vi "gemm_extended_kalman_filter.vi"(8 "Pin":T1, 9 "Uin":dbl[](array[numeric]), 10 "Xin":dbl[](array[numeric]), 11 "Zin":dbl[](array[numeric])) -> (2 "Pout":T1, 3 "Xout":dbl[](array[numeric]))   [LabVIEW 2013]
uses:
  <vilib>/Analysis/Matrix/Datatypes/RealMatrix.ctl
  <vilib>/Analysis/baseanly.llb/A x Vector.vi
  <vilib>/Analysis/baseanly.llb/Real A x B.vi
  <vilib>/Analysis/_algsub.llb/Real PseudoInverse Matrix.vi
  <vilib>/Analysis/BLAS.llb/dgemm - General Matrix-Matrix Product (DBL).vi
  <vilib>/Analysis/NI_AALPro.lvlib
  <vilib>/Analysis/NI_AALBase.lvlib
  <vilib>/Analysis/Matrix/NI_Matrix.lvlib
  <vilib>/Analysis/NI_AALBLAS.lvlib
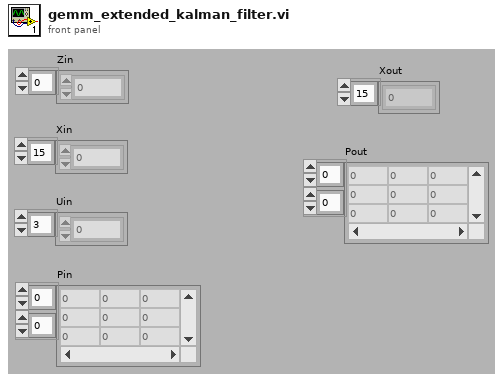
[diagram p1: front panel]
types:
  T1 = typedef "NI_Matrix.lvlib/RealMatrix.ctl" = dbl[][]
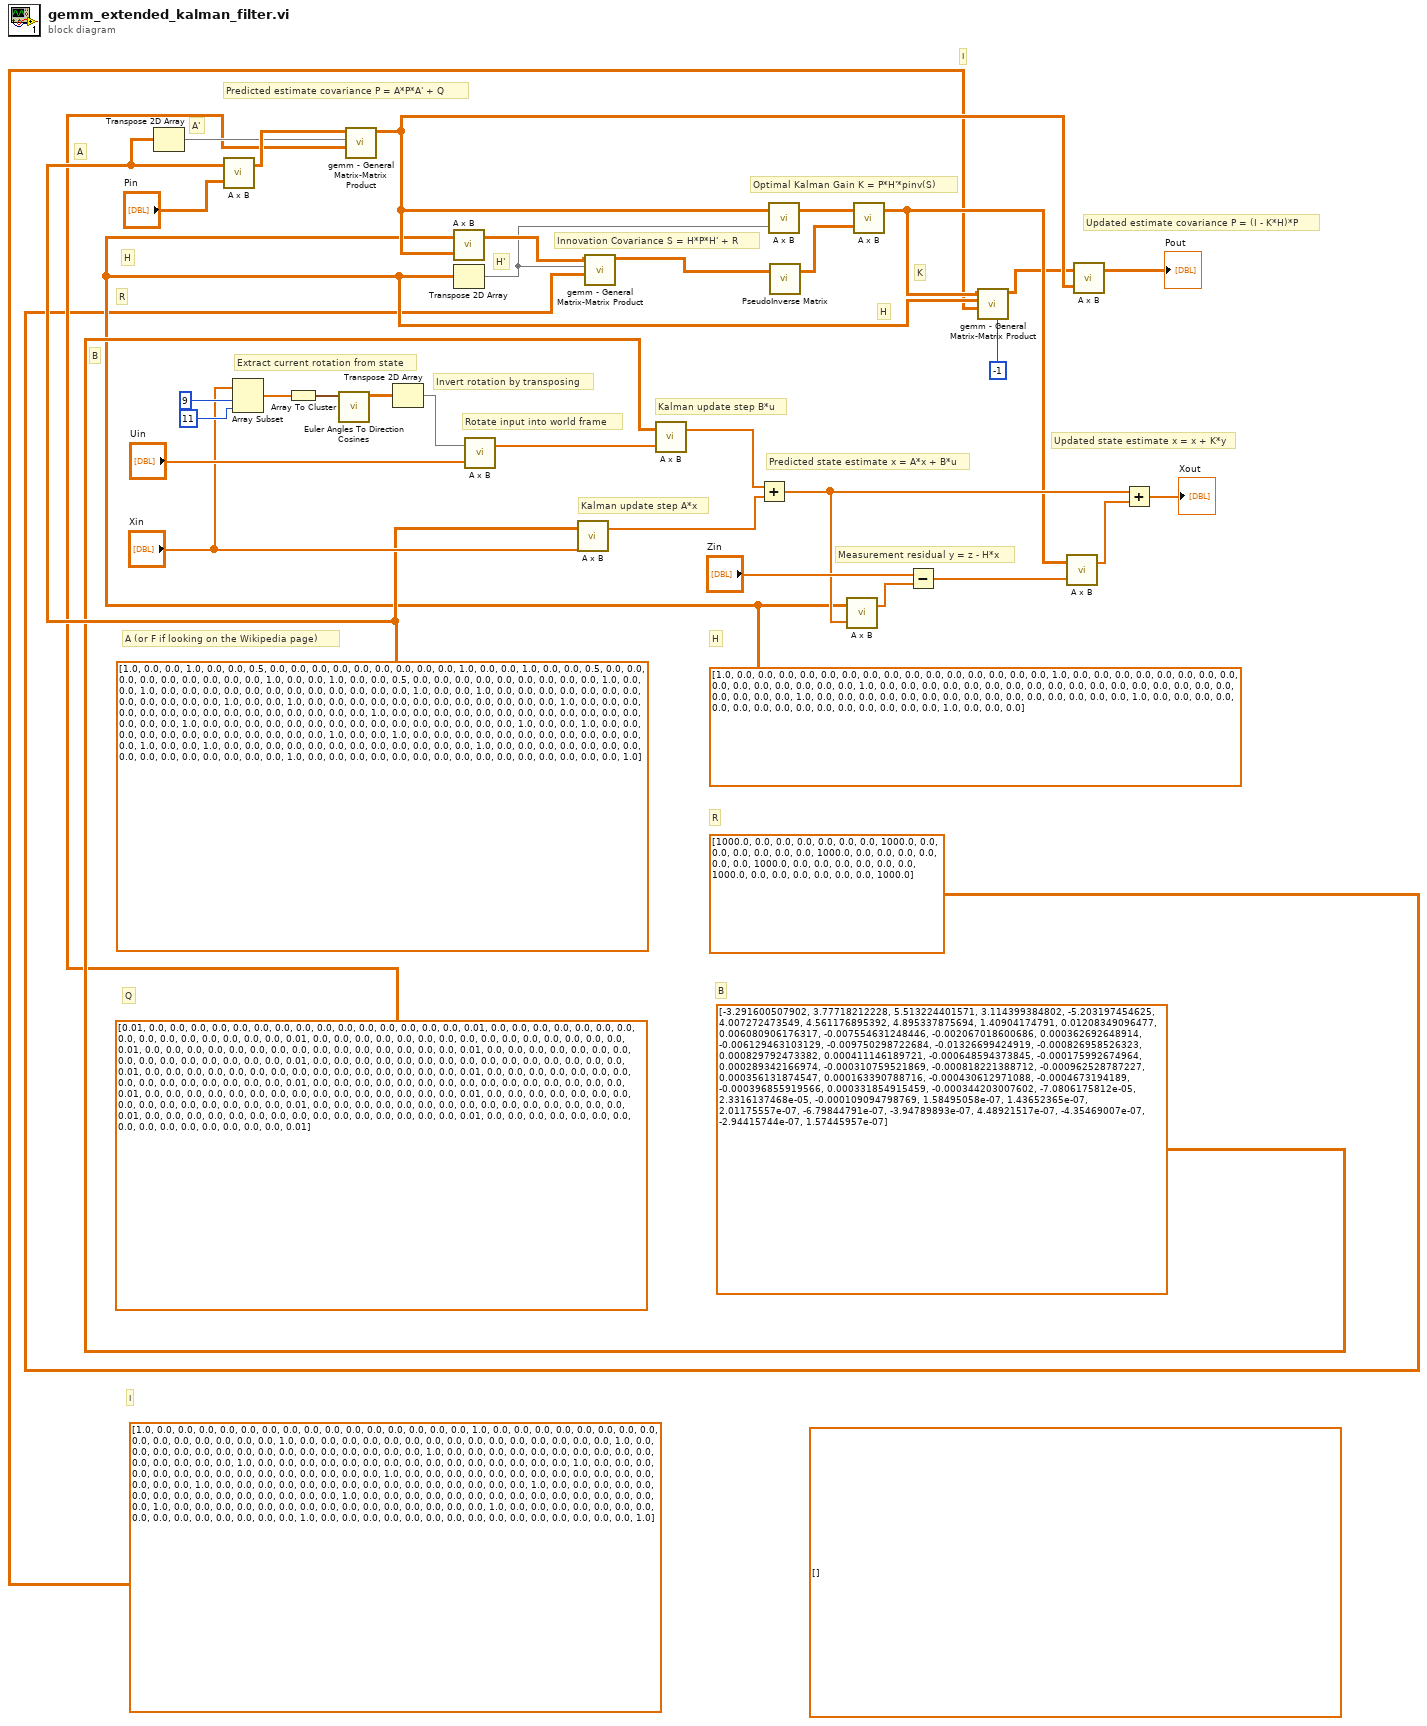
[diagram p0: block diagram]
diagram:
  (unwired) T1 [] ("A + B")
  w8 = T1 [[1.0, 0.0, 0.0, 0.0, 0.0, 0.0, 0.0, 0.0, 0.0, 0.0, 0.0, 0.0, 0.0, 0.0, 0.0], [0.0, 1.0, 0.0, 0.0, 0.0, 0.0, 0.0, 0.0, 0.0, 0.0, 0.0, 0.0, 0.0, 0.0, 0.0], [0.0, 0.0, 1.0, 0.0, 0.0, 0.0, 0.0, 0.0, 0.0, 0.0, 0.0, 0.0, 0.0, 0.0, 0.0], [0.0, 0.0, 0.0, 0.0, 0.0, 0.0, 0.0, 0.0, 0.0, 1.0, 0.0, 0.0, 0.0, 0.0, 0.0], [0.0, 0.0, 0.0, 0.0, 0.0, 0.0, 0.0, 0.0, 0.0, 0.0, 1.0, 0.0, 0.0, 0.0, 0.0], [0.0, 0.0, 0.0, 0.0, 0.0, 0.0, 0.0, 0.0, 0.0, 0.0, 0.0, 1.0, 0.0, 0.0, 0.0]] ("A + B")
  w15 = T1 [[1.0, 0.0, 0.0, 1.0, 0.0, 0.0, 0.5, 0.0, 0.0, 0.0, 0.0, 0.0, 0.0, 0.0, 0.0], [0.0, 1.0, 0.0, 0.0, 1.0, 0.0, 0.0, 0.5, 0.0, 0.0, 0.0, 0.0, 0.0, 0.0, 0.0], [0.0, 0.0, 1.0, 0.0, 0.0, 1.0, 0.0, 0.0, 0.5, 0.0, 0.0, 0.0, 0.0, 0.0, 0.0], [0.0, 0.0, 0.0, 1.0, 0.0, 0.0, 1.0, 0.0, 0.0, 0.0, 0.0, 0.0, 0.0, 0.0, 0.0], [0.0, 0.0, 0.0, 0.0, 1.0, 0.0, 0.0, 1.0, 0.0, 0.0, 0.0, 0.0, 0.0, 0.0, 0.0], [0.0, 0.0, 0.0, 0.0, 0.0, 1.0, 0.0, 0.0, 1.0, 0.0, 0.0, 0.0, 0.0, 0.0, 0.0], [0.0, 0.0, 0.0, 0.0, 0.0, 0.0, 1.0, 0.0, 0.0, 0.0, 0.0, 0.0, 0.0, 0.0, 0.0], [0.0, 0.0, 0.0, 0.0, 0.0, 0.0, 0.0, 1.0, 0.0, 0.0, 0.0, 0.0, 0.0, 0.0, 0.0], [0.0, 0.0, 0.0, 0.0, 0.0, 0.0, 0.0, 0.0, 1.0, 0.0, 0.0, 0.0, 0.0, 0.0, 0.0], [0.0, 0.0, 0.0, 0.0, 0.0, 0.0, 0.0, 0.0, 0.0, 1.0, 0.0, 0.0, 1.0, 0.0, 0.0], [0.0, 0.0, 0.0, 0.0, 0.0, 0.0, 0.0, 0.0, 0.0, 0.0, 1.0, 0.0, 0.0, 1.0, 0.0], [0.0, 0.0, 0.0, 0.0, 0.0, 0.0, 0.0, 0.0, 0.0, 0.0, 0.0, 1.0, 0.0, 0.0, 1.0], [0.0, 0.0, 0.0, 0.0, 0.0, 0.0, 0.0, 0.0, 0.0, 0.0, 0.0, 0.0, 1.0, 0.0, 0.0], [0.0, 0.0, 0.0, 0.0, 0.0, 0.0, 0.0, 0.0, 0.0, 0.0, 0.0, 0.0, 0.0, 1.0, 0.0], [0.0, 0.0, 0.0, 0.0, 0.0, 0.0, 0.0, 0.0, 0.0, 0.0, 0.0, 0.0, 0.0, 0.0, 1.0]] ("A + B")
  # "Updated state estimate x = x + K*y"
  # "Updated estimate covariance P = (I - K*H)*P"
  # "K"
  # "H"
  # "A'"
  # "Invert rotation by transposing"
  # "Measurement residual y = z - H*x"
  # "Optimal Kalman Gain K = P*H'*pinv(S)"
  # "H'"
  # "R"
  # "H"
  # "Innovation Covariance S = H*P*H' + R"
  # "Predicted estimate covariance P = A*P*A' + Q"
  # "B"
  # "A"
  # "I"
  # "Predicted state estimate x = A*x + B*u"
  # "Kalman update step B*u"
  # "Kalman update step A*x"
  # "Rotate input into world frame"
  # "I"
  # "B"
  # "H"
  # "A (or F if looking on the Wikipedia page)"
  # "Extract current rotation from state"
  # "R"
  # "Q"
  n1 = Transpose 2D Array(2D array=w15) -> (transposed array=w12:T1)
  n2 = call-poly <vilib>:"A x B.vi"("B"="Pin", "A"=w15) -> ("A x B"=w13:T1)  [unwired: 1 out]
  n3 = Array Subset(array="Xin", index=9, length=11) -> (w36:dbl[])
  n4 = Array To Cluster(array=w36) -> (cluster=w35:cluster{"[0]":dbl, "[1]":dbl, "[2]":dbl})
  n5 = call <vilib>:"Euler Angles To Direction Cosines.vi"("Euler Angles"=w35) -> ("Direction Cosines"=w32:dbl[][])  [unwired: 9 in, 1 out]
  n6 = call-poly <vilib>:"gemm - General Matrix-Matrix Product.vi"("C"=T1 [[0.01, 0.0, 0.0, 0.0, 0.0, 0.0, 0.0, 0.0, 0.0, 0.0, 0.0, 0.0, 0.0, 0.0, 0.0], [0.0, 0.01, 0.0, 0.0, 0.0, 0.0, 0.0, 0.0, 0.0, 0.0, 0.0, 0.0, 0.0, 0.0, 0.0], [0.0, 0.0, 0.01, 0.0, 0.0, 0.0, 0.0, 0.0, 0.0, 0.0, 0.0, 0.0, 0.0, 0.0, 0.0], [0.0, 0.0, 0.0, 0.01, 0.0, 0.0, 0.0, 0.0, 0.0, 0.0, 0.0, 0.0, 0.0, 0.0, 0.0], [0.0, 0.0, 0.0, 0.0, 0.01, 0.0, 0.0, 0.0, 0.0, 0.0, 0.0, 0.0, 0.0, 0.0, 0.0], [0.0, 0.0, 0.0, 0.0, 0.0, 0.01, 0.0, 0.0, 0.0, 0.0, 0.0, 0.0, 0.0, 0.0, 0.0], [0.0, 0.0, 0.0, 0.0, 0.0, 0.0, 0.01, 0.0, 0.0, 0.0, 0.0, 0.0, 0.0, 0.0, 0.0], [0.0, 0.0, 0.0, 0.0, 0.0, 0.0, 0.0, 0.01, 0.0, 0.0, 0.0, 0.0, 0.0, 0.0, 0.0], [0.0, 0.0, 0.0, 0.0, 0.0, 0.0, 0.0, 0.0, 0.01, 0.0, 0.0, 0.0, 0.0, 0.0, 0.0], [0.0, 0.0, 0.0, 0.0, 0.0, 0.0, 0.0, 0.0, 0.0, 0.01, 0.0, 0.0, 0.0, 0.0, 0.0], [0.0, 0.0, 0.0, 0.0, 0.0, 0.0, 0.0, 0.0, 0.0, 0.0, 0.01, 0.0, 0.0, 0.0, 0.0], [0.0, 0.0, 0.0, 0.0, 0.0, 0.0, 0.0, 0.0, 0.0, 0.0, 0.0, 0.01, 0.0, 0.0, 0.0], [0.0, 0.0, 0.0, 0.0, 0.0, 0.0, 0.0, 0.0, 0.0, 0.0, 0.0, 0.0, 0.01, 0.0, 0.0], [0.0, 0.0, 0.0, 0.0, 0.0, 0.0, 0.0, 0.0, 0.0, 0.0, 0.0, 0.0, 0.0, 0.01, 0.0], [0.0, 0.0, 0.0, 0.0, 0.0, 0.0, 0.0, 0.0, 0.0, 0.0, 0.0, 0.0, 0.0, 0.0, 0.01]] ("A + B"), "B"=w12, "A"=w13) -> ("dgemm"=w10:T1)  [unwired: 7 in, 1 out]
  n7 = Transpose 2D Array(2D array=w32) -> (transposed array=w30:dbl[][])
  n8 = call-poly <vilib>:"A x B.vi"("B"=w10, "A"=w8) -> ("A x B"=w4:T1)  [unwired: 1 out]
  n9 = Transpose 2D Array(2D array=w8) -> (transposed array=w3:T1)
  n10 = call-poly <vilib>:"A x B.vi"("Vector"="Uin", "A"=w30) -> ("A x Vector"=w29:dbl[])  [unwired: 1 out]
  n11 = call-poly <vilib>:"A x B.vi"("Vector"="Xin", "A"=w15) -> ("A x Vector"=w27:dbl[])  [unwired: 1 out]
  n12 = call-poly <vilib>:"gemm - General Matrix-Matrix Product.vi"("C"=T1 [[1000.0, 0.0, 0.0, 0.0, 0.0, 0.0], [0.0, 1000.0, 0.0, 0.0, 0.0, 0.0], [0.0, 0.0, 1000.0, 0.0, 0.0, 0.0], [0.0, 0.0, 0.0, 1000.0, 0.0, 0.0], [0.0, 0.0, 0.0, 0.0, 1000.0, 0.0], [0.0, 0.0, 0.0, 0.0, 0.0, 1000.0]] ("A + B"), "B"=w3, "A"=w4) -> ("dgemm"=w1:T1)  [unwired: 7 in, 1 out]
  n13 = call-poly <vilib>:"A x B.vi"("Vector"=w29, "A"=T1 [[-3.291600507902, 3.77718212228, 5.513224401571], [3.114399384802, -5.203197454625, 4.007272473549], [4.561176895392, 4.895337875694, 1.40904174791], [0.01208349096477, 0.006080906176317, -0.007554631248446], [-0.002067018600686, 0.000362692648914, -0.006129463103129], [-0.009750298722684, -0.01326699424919, -0.000826958526323], [0.000829792473382, 0.000411146189721, -0.000648594373845], [-0.000175992674964, 0.000289342166974, -0.000310759521869], [-0.000818221388712, -0.000962528787227, 0.000356131874547], [0.000163390788716, -0.000430612971088, -0.0004673194189], [-0.000396855919566, 0.000331854915459, -0.000344203007602], [-7.0806175812e-05, 2.3316137468e-05, -0.000109094798769], [1.58495058e-07, 1.43652365e-07, 2.01175557e-07], [-6.79844791e-07, -3.94789893e-07, 4.48921517e-07], [-4.35469007e-07, -2.94415744e-07, 1.57445957e-07]] ("A + B")) -> ("A x Vector"=w28:dbl[])  [unwired: 1 out]
  n14 = Add(x=w28, y=w27) -> (x+y=w20:dbl[])
  n15 = call-poly <vilib>:"A x B.vi"("B"=w3, "A"=w10) -> ("A x B"=w22:T1)  [unwired: 1 out]
  n16 = call-poly <vilib>:"PseudoInverse Matrix.vi"("Input Matrix"=w1) -> ("PseudoInverse Matrix"=w21:T1)  [unwired: 1 in, 1 out]
  n17 = call-poly <vilib>:"A x B.vi"("Vector"=w20, "A"=w8) -> ("A x Vector"=w24:dbl[])  [unwired: 1 out]
  n18 = call-poly <vilib>:"A x B.vi"("B"=w21, "A"=w22) -> ("A x B"=w9:T1)  [unwired: 1 out]
  n19 = Subtract ("Subtract.vi")(x="Zin", y=w24) -> (x-y=w19:dbl[])
  n20 = call-poly <vilib>:"gemm - General Matrix-Matrix Product.vi"("beta"=-1, "C"=T1 [[1.0, 0.0, 0.0, 0.0, 0.0, 0.0, 0.0, 0.0, 0.0, 0.0, 0.0, 0.0, 0.0, 0.0, 0.0], [0.0, 1.0, 0.0, 0.0, 0.0, 0.0, 0.0, 0.0, 0.0, 0.0, 0.0, 0.0, 0.0, 0.0, 0.0], [0.0, 0.0, 1.0, 0.0, 0.0, 0.0, 0.0, 0.0, 0.0, 0.0, 0.0, 0.0, 0.0, 0.0, 0.0], [0.0, 0.0, 0.0, 1.0, 0.0, 0.0, 0.0, 0.0, 0.0, 0.0, 0.0, 0.0, 0.0, 0.0, 0.0], [0.0, 0.0, 0.0, 0.0, 1.0, 0.0, 0.0, 0.0, 0.0, 0.0, 0.0, 0.0, 0.0, 0.0, 0.0], [0.0, 0.0, 0.0, 0.0, 0.0, 1.0, 0.0, 0.0, 0.0, 0.0, 0.0, 0.0, 0.0, 0.0, 0.0], [0.0, 0.0, 0.0, 0.0, 0.0, 0.0, 1.0, 0.0, 0.0, 0.0, 0.0, 0.0, 0.0, 0.0, 0.0], [0.0, 0.0, 0.0, 0.0, 0.0, 0.0, 0.0, 1.0, 0.0, 0.0, 0.0, 0.0, 0.0, 0.0, 0.0], [0.0, 0.0, 0.0, 0.0, 0.0, 0.0, 0.0, 0.0, 1.0, 0.0, 0.0, 0.0, 0.0, 0.0, 0.0], [0.0, 0.0, 0.0, 0.0, 0.0, 0.0, 0.0, 0.0, 0.0, 1.0, 0.0, 0.0, 0.0, 0.0, 0.0], [0.0, 0.0, 0.0, 0.0, 0.0, 0.0, 0.0, 0.0, 0.0, 0.0, 1.0, 0.0, 0.0, 0.0, 0.0], [0.0, 0.0, 0.0, 0.0, 0.0, 0.0, 0.0, 0.0, 0.0, 0.0, 0.0, 1.0, 0.0, 0.0, 0.0], [0.0, 0.0, 0.0, 0.0, 0.0, 0.0, 0.0, 0.0, 0.0, 0.0, 0.0, 0.0, 1.0, 0.0, 0.0], [0.0, 0.0, 0.0, 0.0, 0.0, 0.0, 0.0, 0.0, 0.0, 0.0, 0.0, 0.0, 0.0, 1.0, 0.0], [0.0, 0.0, 0.0, 0.0, 0.0, 0.0, 0.0, 0.0, 0.0, 0.0, 0.0, 0.0, 0.0, 0.0, 1.0]] ("A + B"), "B"=w8, "A"=w9) -> ("dgemm"=w6:T1)  [unwired: 6 in, 1 out]
  n21 = call-poly <vilib>:"A x B.vi"("Vector"=w19, "A"=w9) -> ("A x Vector"=w18:dbl[])  [unwired: 1 out]
  n22 = call-poly <vilib>:"A x B.vi"("B"=w10, "A"=w6) -> ("A x B"=→"Pout":T1)  [unwired: 1 out]
  n23 = Add(x=w20, y=w18) -> (x+y=→"Xout":dbl[])
